vi "New Results (to override).vi"(7 "Image Nr.":i32, 8 "error in (no error)":errorcluster, 9 "Results In":refnum<class "Analyze Results Base.lvclass">[](array[class]), 10 "Parameters":refnum<class "Analyze Parameter Base.lvclass">[](array[class]), 11 "Launch IMAQ Display in":refnum<class "HIJ Vision Application.lvclass">) -> (0 "error out":errorcluster, 3 "Launch IMAQ Display out":refnum<class "HIJ Vision Application.lvclass">)   [LabVIEW 2020]
uses:
  HIJ Vision Application.lvclass
  Analyze/Results and Overlays/Results Base/Analyze Results Base.lvclass
  Analyze/Analyze Parameter/Analyze Parameter Base/Analyze Parameter Base.lvclass
  HIJ Vision Application.lvclass/HIJ Vision Application.ctl
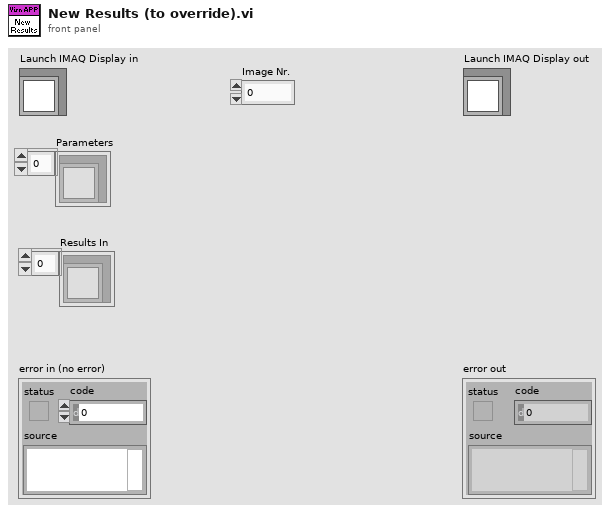
[diagram p1: front panel]
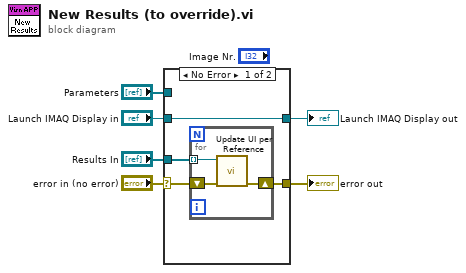
[diagram p0: block diagram]
diagram:
  n1 = case shown="No Error" "error in (no error)" {
    selector: "error in (no error)" -> [w8 w15]
    tunnel: [w7 w15] -> w5
    tunnel: [w10 w14] -> w3
    tunnel: "Launch IMAQ Display in" -> [w10 w14]
    tunnel: "Parameters" -> [_ _]
    tunnel: "Results In" -> [w9 _]
    frame No Error {
      n2 = for {
        tunnel: w9 -> [w13] mode=indexing
        shift-right: [w11] -> w7
        shift-left: w8 -> [w12]
        n3 = call-dynamic "Update UI per Reference.vi"("error in (no error)"=w12, "Analyze Results Base in"=w13) -> ("error out"=w11:errorcluster)  [unwired: 8 in, 1 out]
      }
    }
    frame Error {
    }
  }
  "error out" <- w5
  "Launch IMAQ Display out" <- w3
